vi "locate system variable in configuration.vi"(8 "error in":errorcluster, 10 "raw variable data":T1, 11 "Scan Engine configuration in":refnum<class "Scan Engine configuration.lvclass">) -> (0 "error out":errorcluster, 1 "found?":bool, 2 "channel":refnum<class "TBM channel.lvclass">, 3 "Scan Engine configuration out":refnum<class "Scan Engine configuration.lvclass">)   [LabVIEW 2014, in "Scan Engine runtime.lvclass"]
uses:
  Scan Engine runtime.lvclass
  <vilib>/NI/Tag Bus Module Framework/channel/TBM channel.lvclass
  configuration/Scan Engine configuration.lvclass
  Custom Ctrls/system variable.ctl
  <vilib>/NI/Tag Bus/tag/Data Type.ctl
  <vilib>/NI/Tag Bus/tag/tag descriptor.lvclass/tag descriptor.ctl
  <vilib>/NI/Tag Bus/tag/read tag name.vi
  <resource>/objmgr/ni.var.rc
  <vilib>/NI/Tag Bus/tag/tag descriptor.lvclass
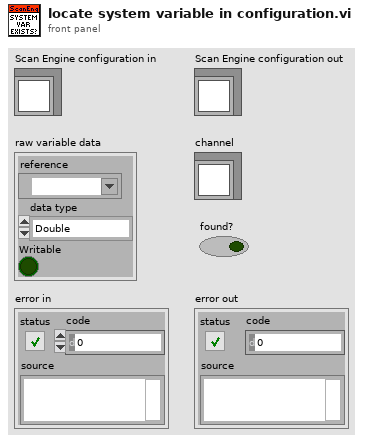
[diagram p1: front panel]
types:
  T1 = typedef "Scan Engine runtime.lvclass/system variable.ctl" = cluster{"reference":refnum<k21>, "data type":T2, "Writable":bool}
  T2 = typedef "tag bus.lvlib/tag descriptor.lvclass/Data Type.ctl" = enum16{"Double", "Single", "I64", "I32", "I16", "I8", "U64", "U32", "U16", "U8", "Boolean", "String", "Array of Double", "Array of Single", "Array of I64", "Array of I32", "Array of I16", "Array of I8", "Array of U64", "Array of U32", "Array of U16", "Array of U8", "Array of Boolean", "Array of String"}
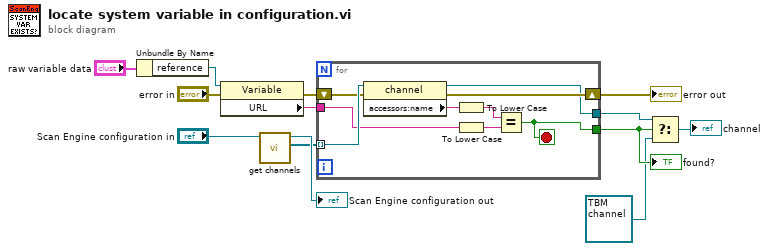
[diagram p0: block diagram]
diagram:
  n1 = Unbundle By Name("raw variable data") -> ("reference"=w11:refnum<k21>)
  n2 = property class="Variable"(reference=w11, error in="error in") -> (error out=w1:errorcluster, "URL"=w9:string)  [unwired: 1 out]
  n3 = call-dynamic "get channels.vi"("Scan Engine configuration in"="Scan Engine configuration in") -> ("channels"=w2:refnum<class "TBM channel.lvclass">[], "Scan Engine configuration out"=→"Scan Engine configuration out":refnum<class "Scan Engine configuration.lvclass">)  [unwired: 9 in]
  n4 = for {
    tunnel: w2 -> [w22] mode=indexing
    shift-right: [w16] -> w7
    shift-left: w1 -> [w21]
    tunnel: w9 -> [w20]
    tunnel: [w15] -> w5
    tunnel: [w14] -> w6
    stop <- w14 stop-if-true
    n5 = property class="channel"(reference=w22, error in=w21) -> (reference out=w15:refnum<class "TBM channel.lvclass">, error out=w16:errorcluster, "accessors:name"=w19:string)
    n6 = To Lower Case(string=w19) -> (all lower case string=w18:string)
    n7 = To Lower Case(string=w20) -> (all lower case string=w17:string)
    n8 = Equal?(x=w18, y=w17) -> (x = y?=w14:bool)
  }
  "found?" <- w6
  "error out" <- w7
  n9 = Select(t=w5, s=w6, f=refnum<class "TBM channel.lvclass"> refnum) -> (s? t:f=→"channel":refnum<class "TBM channel.lvclass">)
